vi "Unflatten U32.vi"(3 "Flat Data":u8[](array[numeric]) format="%.0x", 4 "Endian":T1) -> (5 "U32":u32 format="%.0x")   [LabVIEW 2021, in "DataTypes_CIF_U.lvlib"]
uses:
  DataTypes_CIF_U.lvlib
  Endian.ctl
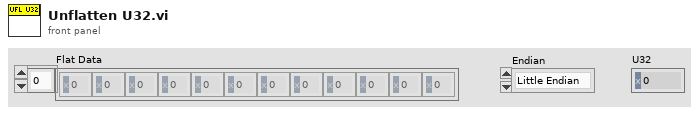
[diagram p1: front panel]
types:
  T1 = typedef "DataTypes_CIF_U.lvlib/Endian.ctl" = enum16{"Little Endian", "Big Endian"}
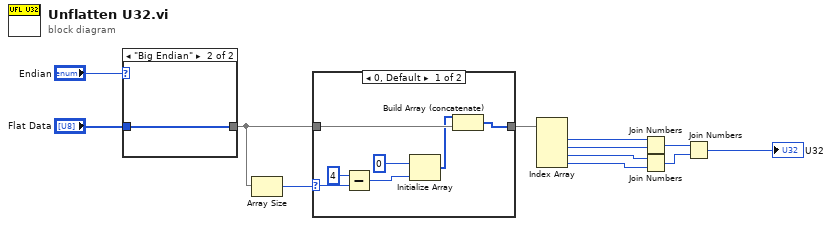
[diagram p0: block diagram]
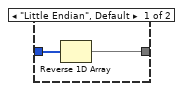
[diagram p3: hidden frame]
diagram:
  n1 = case shown="\"Big Endian\"" "Endian" {
    tunnel: "Flat Data" -> [w14 w15]
    tunnel: [w13 w15] -> w2
    frame "Little Endian", Default {
      n2 = Reverse 1D Array(array=w14) -> (reversed array=w13:u8[])
    }
    frame "Big Endian" {
    }
  }
  n3 = Array Size(array=w2) -> (size(s)=w5:i32)
  n4 = case shown="0, Default" w5 {
    selector: w5 -> [w22 _]
    tunnel: w2 -> [w18 w23]
    tunnel: [w16 w23] -> w3
    frame 0, Default {
      n5 = Subtract(x=4, y=w22) -> (x-y=w19:i32)
      n6 = Initialize Array(u8 0 ("element"), w19) -> (w17:u8[])
      n7 = Build Array (concatenate)(w17, w18) -> (w16:u8[])
    }
    frame 4.. {
    }
  }
  n8 = Index Array(array=w3) -> (element #1=w11:u8, element #2=w8:u8, element #3=w7:u8, element #4=w6:u8)  [unwired: 4 in]
  n9 = Join Numbers(hi=w11, lo=w8) -> ((hi.lo)=w10:u16)
  n10 = Join Numbers(hi=w7, lo=w6) -> ((hi.lo)=w9:u16)
  n11 = Join Numbers(hi=w10, lo=w9) -> ((hi.lo)=→"U32":u32)
